vi "Newmark-JogLinear.vi"(0 "Table VRN IN":refnum<visa-resource-name>="COM9", 2 "Bool Refnum":refnum<vi>, 11 "Error IN":errorcluster, 12 "Position X":dbl, 13 "Position Y":dbl, 14 "Vitesse Jog":dbl) -> (4 "Table VRN OUT":refnum<visa-resource-name>="COM9", 15 "Error OUT":errorcluster)   [LabVIEW 2019]
uses:
  Comm/SerialCommError.vi
panel:
  out "Command Line":string
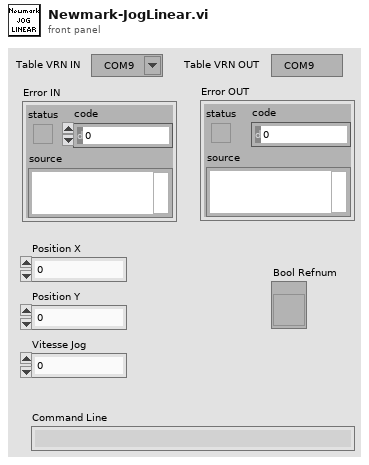
[diagram p1: front panel]
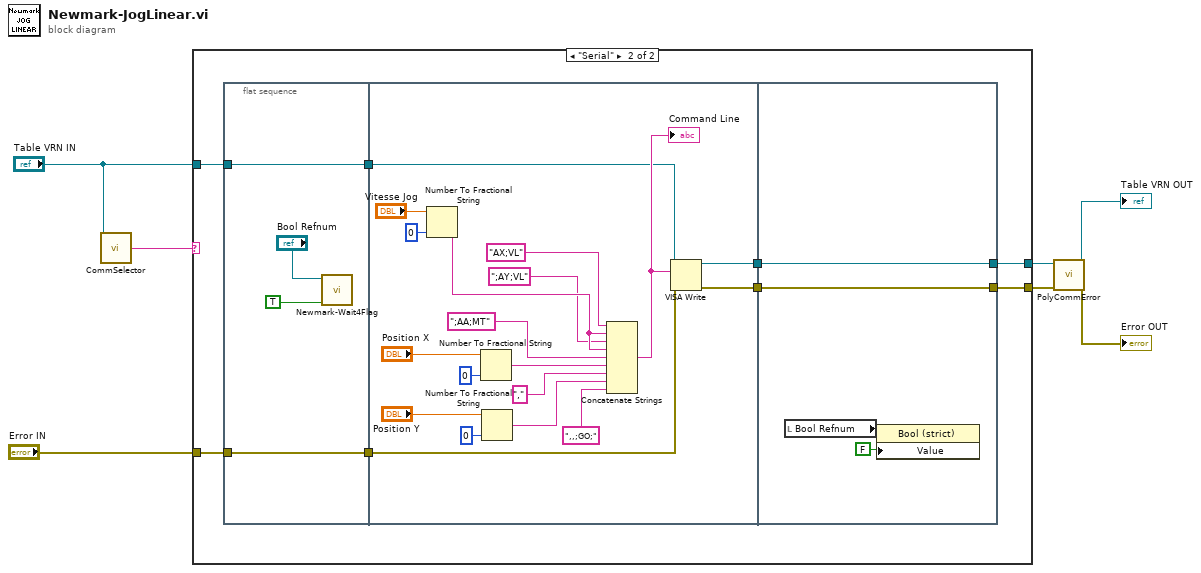
[diagram p0: block diagram]
diagram:
  n1 = call "CommSelector.vi"("VISA resource name"="Table VRN IN") -> ("CommType"=w1:string)  [unwired: 13 in, 1 out]
  n2 = case shown="\"Serial\"" w1 {
    tunnel: "Table VRN IN" -> [w9 w16]
    tunnel: "Error IN" -> [w8 w14]
    tunnel: [w9 w13] -> w6
    tunnel: [w8 w11] -> w7
    frame "Unknown", Default {
    }
    frame "Serial" {
      n3 = flat-sequence {
        tunnel: [w19] -> w17
        tunnel: w16 -> [w19]
        tunnel: [w18] -> w15
        tunnel: w14 -> [w18]
        tunnel: w17 -> [w35]
        tunnel: w15 -> [w34]
        tunnel: [w33] -> w12
        tunnel: [w32] -> w10
        tunnel: [w42] -> w13
        tunnel: w12 -> [w42]
        tunnel: [w41] -> w11
        tunnel: w10 -> [w41]
        frame #0 {
          n4 = call "Newmark-Wait4Flag.vi"("Raise Flag ?"=TRUE, "Ctl Refnum IN"="Bool Refnum") -> ()  [unwired: 8 in, 2 out]
        }
        frame #1 {
          n5 = Number To Fractional String(number="Vitesse Jog", precision (6)=i16 0) -> (F-format string=w23:string)  [unwired: 2 in]
          n6 = Number To Fractional String(number="Position X", precision (6)=i16 0) -> (F-format string=w37:string)  [unwired: 2 in]
          n7 = Number To Fractional String(number="Position Y", precision (6)=i16 0) -> (F-format string=w30:string)  [unwired: 2 in]
          n8 = Concatenate Strings("AX;VL" ("string"), w23, ";AY;VL" ("string"), w23, ";AA;MT" ("string"), w37, "," ("string"), w30, ",,;GO;" ("string")) -> (w39:string)
          "Command Line" <- w39
          n9 = VISA Write(VISA resource name=w35, write buffer=w39, error in (no error)=w34) -> (VISA resource name out=w33:refnum<visa-resource-name>, error out=w32:errorcluster)  [unwired: 1 out]
        }
        frame #2 {
          n10 = local read "Bool Refnum"() -> (w44:refnum<vi>)
          n11 = property class="Bool (strict)"(reference=w44, "Value"=FALSE) -> ()  [unwired: 1 in, 2 out]
        }
      }
    }
  }
  n12 = call-poly "PolyCommError.vi"("VISA IN"=w6, "error IN"=w7) -> ("VISA OUT"=→"Table VRN OUT":refnum<visa-resource-name>, "error OUT"=→"Error OUT":errorcluster)  [unwired: 11 in, 1 out]
